vi "Debug Exercise (Main).vi"() -> ()   [LabVIEW 2010]
doc: "This VI is part of Exercise 2-3 in the LabVIEW Basics I Course.\n\nFirst, fix the broken run arrow and then use the different debugging tools to see how they work."
panel:
  out "Final Result":dbl format="%.2f"
  out "Random Number":dbl format="%.2f"
  in  "Multiply Result":dbl format="%.2f"
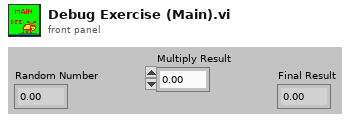
[diagram p1: front panel]
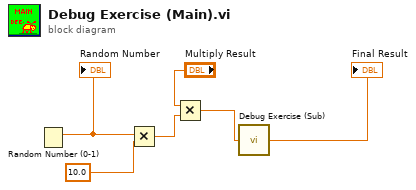
[diagram p0: block diagram]
diagram:
  n1 = Random Number (0-1)() -> (number: 0 to 1=w5:dbl)
  "Random Number" <- w5
  n2 = Multiply(x=w5, y=10.0) -> (x*y=w4:dbl)
  n3 = Multiply(x="Multiply Result", y=w4) -> (x*y=w2:dbl)
  n4 = call "Debug Exercise (Sub).vi"("Number"=w2) -> ("Final Result"=→"Final Result":dbl)
